vi "Ampel.vi"() -> ()   [LabVIEW 2016]
panel:
  in  "Dauer Phase 2":u64 max=120 step=1
  in  "Transitionsphase nach 1":u64 max=120 step=1
  in  "Dauer Phase 1":u64 max=120 step=1
  in  "Trasitionsphase nach 2":u64 max=120 step=1
  out "Ampel2 2":T1
  out "Ampel1 2":T1
  out "Fussg":cluster{"Boolesch":bool, "Boolesch 2":bool}={"Boolesch"=TRUE, "Boolesch 2"=FALSE}
  out "Ampel2":T1
  out "Ampel1":T1
  in  "Fußgänger":bool
  in  "Stopp":bool
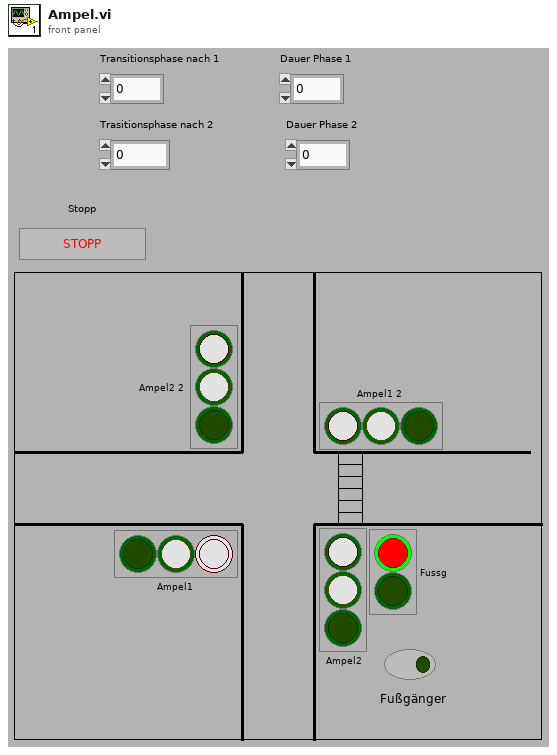
[diagram p1: front panel]
types:
  T1 = cluster{"Boolesch":bool, "Boolesch 2":bool, "Boolesch 3":bool}
  T2 = cluster{"Boolean array[0]":bool, "Boolean array[1]":bool, "Boolean array[2]":bool}
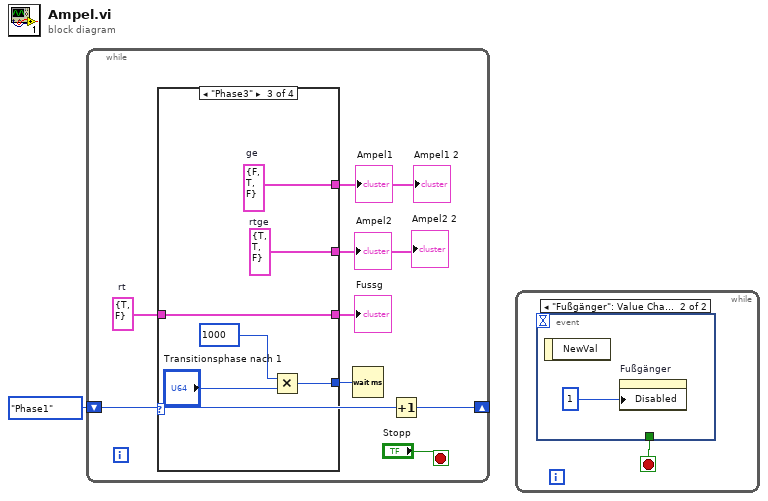
[diagram p0: block diagram]
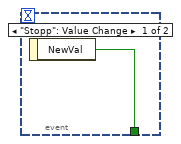
[diagram p2: hidden frame]
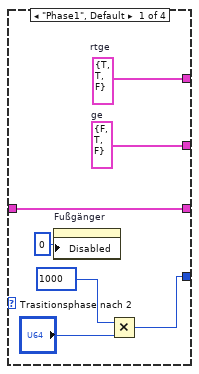
[diagram p3: hidden frame]
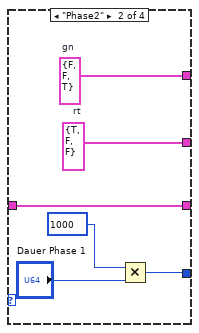
[diagram p4: hidden frame]
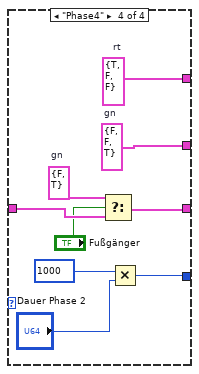
[diagram p5: hidden frame]
diagram:
  n1 = while {
    shift-right: [w3] -> _
    shift-left: enum16{"Phase1", "Phase2", "Phase3", "Phase4"}."Phase1" ("Enum") -> [w2]
    stop <- "Stopp" stop-if-true
    w6 = cluster{"Boolesch":bool, "Boolesch 2":bool} {"Boolesch"=TRUE, "Boolesch 2"=FALSE}  # rt
    n2 = case shown="\"Phase3\"" w2 {
      tunnel: [w16 w22 w28 w36] -> w4
      tunnel: [w15 w21 w27 w37] -> w5
      tunnel: [w10 w17 w25 w29] -> w8
      tunnel: [w14 w20 w26 w35] -> w7
      tunnel: w6 -> [w14 w20 w26 w34]
      frame "Phase1", Default {
        w15 = T2 {"Boolean array[0]"=FALSE, "Boolean array[1]"=TRUE, "Boolean array[2]"=FALSE}  # ge
        w16 = T2 {"Boolean array[0]"=TRUE, "Boolean array[1]"=TRUE, "Boolean array[2]"=FALSE}  # rtge
        n3 = property on="Fußgänger" class="Bool"("Disabled"=u8 0 ("Deaktiviert")) -> ()  [unwired: 2 in, 2 out]
        n4 = Multiply(x=u64 1000, y="Trasitionsphase nach 2") -> (x*y=w10:u64)
      }
      frame "Phase2" {
        w21 = T2 {"Boolean array[0]"=TRUE, "Boolean array[1]"=FALSE, "Boolean array[2]"=FALSE}  # rt
        w22 = T2 {"Boolean array[0]"=FALSE, "Boolean array[1]"=FALSE, "Boolean array[2]"=TRUE}  # gn
        n5 = Multiply(x=u64 1000, y="Dauer Phase 1") -> (x*y=w17:u64)
      }
      frame "Phase3" {
        w27 = T2 {"Boolean array[0]"=TRUE, "Boolean array[1]"=TRUE, "Boolean array[2]"=FALSE}  # rtge
        w28 = T2 {"Boolean array[0]"=FALSE, "Boolean array[1]"=TRUE, "Boolean array[2]"=FALSE}  # ge
        n6 = Multiply(x=u64 1000, y="Transitionsphase nach 1") -> (x*y=w25:u64)
      }
      frame "Phase4" {
        w33 = cluster{"Boolesch":bool, "Boolesch 2":bool} {"Boolesch"=FALSE, "Boolesch 2"=TRUE}  # gn
        w36 = T2 {"Boolean array[0]"=TRUE, "Boolean array[1]"=FALSE, "Boolean array[2]"=FALSE}  # rt
        w37 = T2 {"Boolean array[0]"=FALSE, "Boolean array[1]"=FALSE, "Boolean array[2]"=TRUE}  # gn
        n7 = Select(t=w33, s="Fußgänger", f=w34) -> (s? t:f=w35:cluster{"Boolesch":bool, "Boolesch 2":bool})
        n8 = Multiply(x=u64 1000, y="Dauer Phase 2") -> (x*y=w29:u64)
      }
    }
    "Ampel1" <- w4
    "Ampel2" <- w5
    "Fussg" <- w7
    "Ampel1 2" <- w4
    "Ampel2 2" <- w5
    n9 = Wait (ms)(milliseconds to wait=w8) -> ()  [unwired: 1 out]
    n10 = Increment(x=w2) -> (x+1=w3:enum16{"Phase1", "Phase2", "Phase3", "Phase4"})
  }
  n11 = while {
    stop <- w38 stop-if-true
    n12 = event shown="[1] \"Fußgänger\": Value Change" {
      selector: _ -> [_ _]
      dyn-events: _ -> [_ _]
      timeout: _ -> [_ _]
      tunnel: [w39 _] -> w38
      event "Stopp": Value Change {
        n13 = event-data() -> ("NewVal"=w39:bool)  [unwired: 1 out]
      }
      event "Fußgänger": Value Change {
        n14 = event-data() -> ()  [unwired: 2 out]
        n15 = property on="Fußgänger" class="Bool"("Disabled"=u8 1 ("Deaktiviert")) -> ()  [unwired: 2 in, 2 out]
      }
    }
  }
